vi "ProcessVIsNames.vi"(8 "error in (no error)":errorcluster, 11 "VIs":refnum<vi>[](array[refnum])) -> (0 "error out":errorcluster, 2 "VIsData":T1[](array[typedef]), 3 "VIs out":refnum<vi>[](array[refnum]))   [LabVIEW 2020]
uses:
  _controls/_VIWiresData.ctl
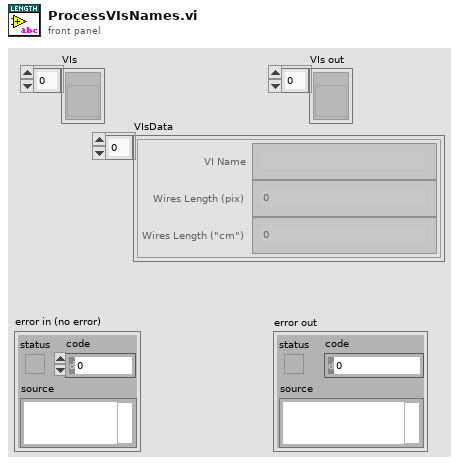
[diagram p1: front panel]
types:
  T1 = typedef "_VIWiresData.ctl" = cluster{"VI Name":string, "Wires Length (pix)":dbl, "Wires Length (\"cm\")":dbl}
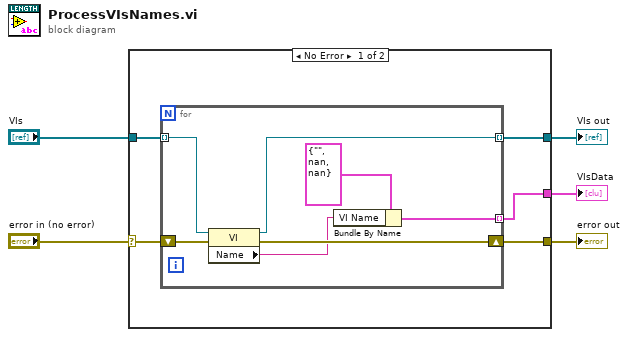
[diagram p0: block diagram]
diagram:
  n1 = case shown="No Error" "error in (no error)" {
    selector: "error in (no error)" -> [w9 w19]
    tunnel: [w8 w19] -> w5
    tunnel: [w7 w18] -> w3
    tunnel: "VIs" -> [w10 w18]
    tunnel: [w6 _] -> w1
    frame No Error {
      n2 = for {
        tunnel: w10 -> [w15] mode=indexing
        shift-right: [w16] -> w8
        shift-left: w9 -> [w17]
        tunnel: [w14] -> w7 mode=indexing
        tunnel: [w11] -> w6 mode=indexing
        n3 = property class="VI"(reference=w15, error in=w17) -> (reference out=w14:refnum<vi>, error out=w16:errorcluster, "Name"=w12:string)
        n4 = Bundle By Name(cluster=T1 {"VI Name"="", "Wires Length (pix)"=nan, "Wires Length (\"cm\")"=nan} ("VIWiresData"), "VI Name"=w12) -> (w11:T1)
      }
    }
    frame Error {
    }
  }
  "error out" <- w5
  "VIs out" <- w3
  "VIsData" <- w1
